vi "_Last Sibling or Self.vi"(8 "error in (no error)":errorcluster, 11 "NodeRef In":refnum<data-value>) -> (0 "error out":errorcluster, 2 "Last Sibling or Self":refnum<data-value>, 3 "NodeRef":refnum<data-value>)   [LabVIEW 2020]
uses:
  Node.lvclass
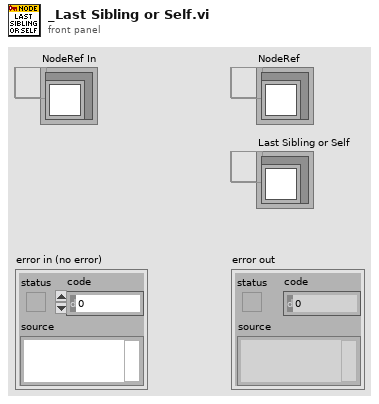
[diagram p1: front panel]
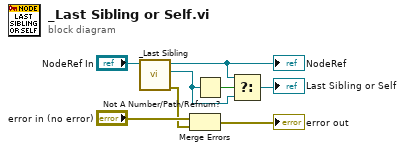
[diagram p0: block diagram]
diagram:
  n1 = call "_Last Sibling.vi"("NodeRef In"="NodeRef In") -> ("error out"=w1:errorcluster, "Last Sibling"=w5:refnum<data-value>, "NodeRef"=w4:refnum<data-value>)  [unwired: 8 in]
  "NodeRef" <- w4
  n2 = Merge Errors("error in (no error)", w1) -> (→"error out":errorcluster)
  n3 = Not A Number/Path/Refnum?(number/path/refnum=w5) -> (NaN/Path/Refnum?=w6:bool)
  n4 = Select(t=w4, s=w6, f=w5) -> (s? t:f=→"Last Sibling or Self":refnum<data-value>)
